vi "Parse Data for Logging.vi"(11 "Instrument State":T1) -> (3 "Array":string[](array[string]))   [LabVIEW 2020, in "Deep Reaction Optimizer Control Panel.lvlib" / "Logging.lvlib"]
doc: "Parses the Instrument State typedef data into an array of strings to be written to a log file."
uses:
  Logging.lvlib
  Instrument Manager/Instrument State.ctl
  <vilib>/addons/zeromq/zmq_context.lvclass
  <vilib>/addons/zeromq/zmq_socket.lvclass
  Instrument Manager/Instrument Manager.lvlib
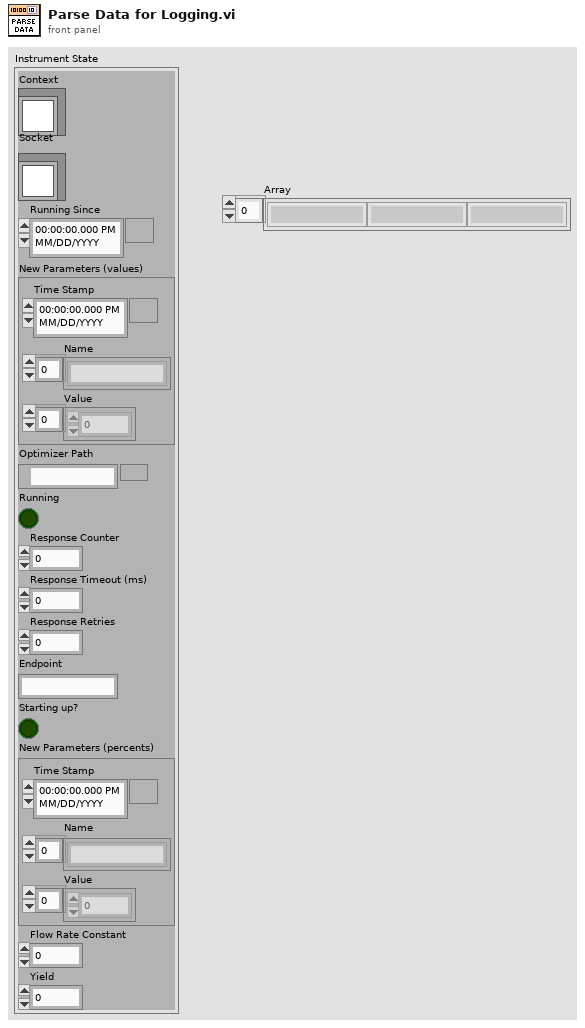
[diagram p1: front panel]
types:
  T1 = typedef "Deep Reaction Optimizer Control Panel.lvlib/Instrument Manager.lvlib/Instrument State.ctl" = cluster{"Context":refnum<class "zmq_context.lvclass">, "Socket":refnum<class "zmq_socket.lvclass">, "Running Since":timestamp, "New Parameters (values)":cluster{"Time Stamp":timestamp, "Name":string[], "Value":dbl[]}, "Optimizer Path":path, "Running":bool, "Response Counter":u8, "Response Timeout (ms)":u32, "Response Retries":u32, "Endpoint":string, "Starting up?":bool, "New Parameters (percents)":cluster{"Time Stamp":timestamp, "Name":string[], "Value":dbl[]}, "Flow Rate Constant":dbl, "Yield":dbl}
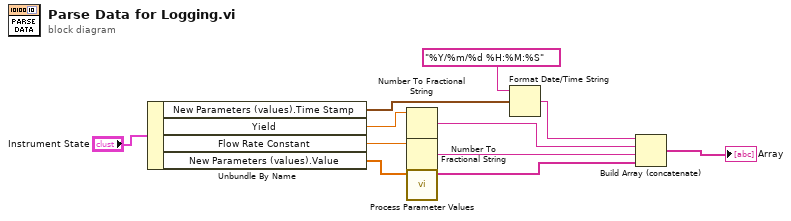
[diagram p0: block diagram]
diagram:
  n1 = Unbundle By Name("Instrument State") -> ("New Parameters (values).Time Stamp"=w10:timestamp, "Yield"=w2:dbl, "Flow Rate Constant"=w5:dbl, "New Parameters (values).Value"=w6:dbl[])
  n2 = Number To Fractional String(number=w2) -> (F-format string=w1:string)  [unwired: 3 in]
  n3 = Number To Fractional String(number=w5) -> (F-format string=w4:string)  [unwired: 3 in]
  n4 = call "Process Parameter Values.vi"("Parameter Values"=w6) -> ("Processed Parameter Value Strings"=w7:string[])  [unwired: 10 in]
  n5 = Format Date/Time String(time format string (%c)="%Y/%m/%d %H:%M:%S", seconds (now)=w10) -> (date/time string=w3:string)  [unwired: 1 in]
  n6 = Build Array (concatenate)(w3, w1, w4, w7) -> (→"Array":string[])
